vi "Connect Terminals.vi"(8 "error in (no error)":errorcluster, 9 "Sink":string, 10 "Source":string, 11 "map":map{string, refnum<vi>}(c390)) -> (0 "error out":errorcluster)   [LabVIEW 2020, in "Pure Mock Class Generator.lvclass"]
uses:
  Pure Mock Class Generator.lvclass
panel:
  out "map 2":map{string, refnum<vi>}(c390)
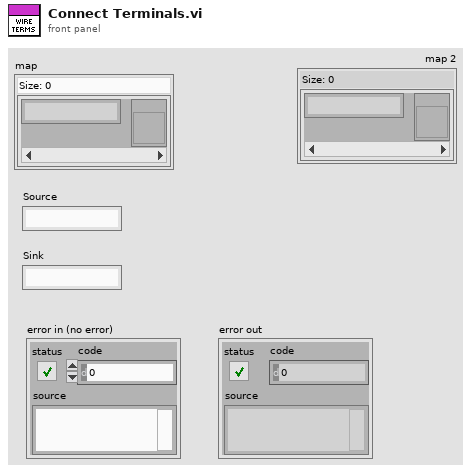
[diagram p1: front panel]
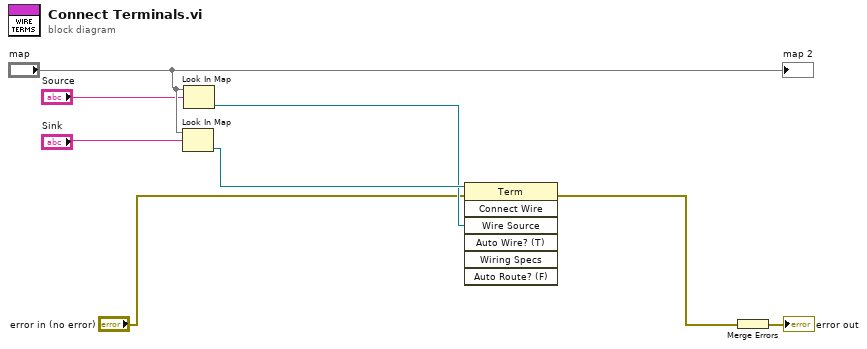
[diagram p0: block diagram]
diagram:
  n1 = Look In Map(map="map", key="Sink") -> (value=w4:refnum<vi>)  [unwired: 1 in, 1 out]
  n2 = Look In Map(map="map", key="Source") -> (value=w3:refnum<vi>)  [unwired: 1 in, 1 out]
  n3 = invoke class="Term" method="Connect Wire"(reference=w4, error in="error in (no error)", "Wire Source"=w3) -> (error out=w1:errorcluster)  [unwired: 4 in, 6 out]
  n4 = Merge Errors(w1) -> (→"error out":errorcluster)
  "map 2" <- "map"
